vi "HB_ImaqAttributeTree.vi"() -> ()   [LabVIEW 2009, in "HB_IMAQ_Examples.lvlib"]
doc: "The HL Snap VI acquires an image and displays the image in an image control using the high-level acquisition VIs. A snap is appropriate for low-speed or single-capture applications where ease of programming is essential.\n\nIMAQ Init initializes the device. IMAQ Create creates an image buffer. IMAQ Snap acquires an image into the buffer, and an image control displays the image on the front panel. IMAQ Close releases resources associated with the acquisition, and the IMAQ Dispose frees the image buffer. Use this sequence to ensure that the image control displays the image before the memory is disposed."
uses:
  HB_IMAQ_Examples.lvlib
  <vilib>/vision/driver/IMAQdx.llb/IMAQdx Attribute Type.ctl
  lib.lib/HGF_LVC/HGF_IMAQ/HGF_IMAQFactory/HGF_IMAQFactory.lvclass
  lib.lib/HGF_LVC/HGF_IMAQ/HGF_IMAQDevice/HGF_IMAQDevice.lvclass
  lib.lib/HGF_LVC/HGF_BaseClasses/HGF_Factory/HGF_Factory.lvclass
  lib.lib/HGF_LVC/HGF_DeviceBaseClasses/HGF_DeviceBase/HGF_DeviceBase.lvclass
  lib.lib/HGF_LVC/HGF_Auxiliary/HGF_Auxiliary.lvlib
  <vilib>/vision/driver/NI_Vision_Acquisition_Software.lvlib
panel:
  out "Units":string
  out "Tooltip":string
  in  "Attribute Tab Control":T1(tab)
  in  "U32 Value Control":u32(slide) min=1 step=1 scale=1.0..4294967295.0
  in  "DBL Value Control":dbl(slide) min=0.00010395202398217064 max=1000.0 step=1.0 scale=0.00010395202398217064..1000.0
  in  "String Value Control":string
  in  "Enum Value Control":u32(ring) items=["Unicast", "Broadcast", "Multicast"]
  in  "Boolean Value Control":bool=TRUE
  in  "Command Value Control":bool
  in  "Attribute Table":string(tree)
  in  "stop":bool
  out "error out":errorcluster
  out "Attribute Information":T3(array[cluster])
  out "Video Modes":T4(array[cluster])
  in  "cameraName":string="cam0"
  in  "imaqClassName":string="HGF_ImaqDx"
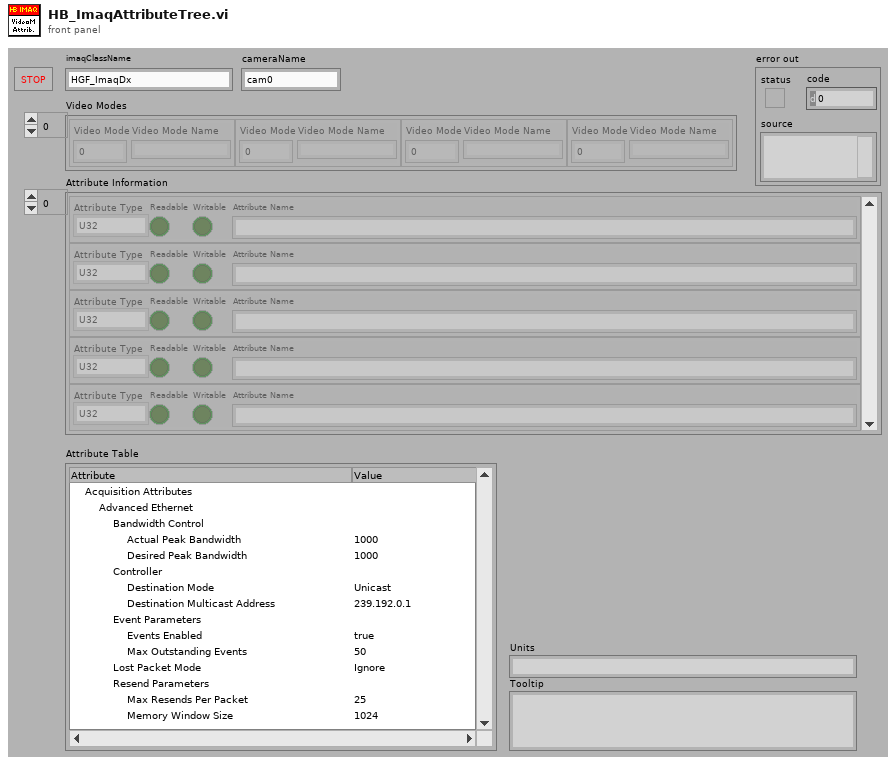
[diagram p1: front panel]
types:
  T1 = enum32{"U32", "DBL", "String", "Enum", "Bool", "Command"}
  T2 = typedef "NI_Vision_Acquisition_Software.lvlib/IMAQdx Attribute Type.ctl" = enum32{"U32", "I64", "DBL", "String", "Enum", "Bool", "Command"}
  T3 = cluster{"Attribute Type":T2, "Readable":bool, "Writable":bool, "Attribute Name":string}[]
  T4 = cluster{"Video Mode":u32, "Video Mode Name":string}[]
  T5 = cluster{"Attribute Tab Control":refnum<vi>, "U32 Value Control":refnum<vi>, "DBL Value Control":refnum<vi>, "String Value Control":refnum<vi>, "Enum Value Control":refnum<vi>, "Boolean Value Control":refnum<vi>, "Command Value Control":refnum<vi>}
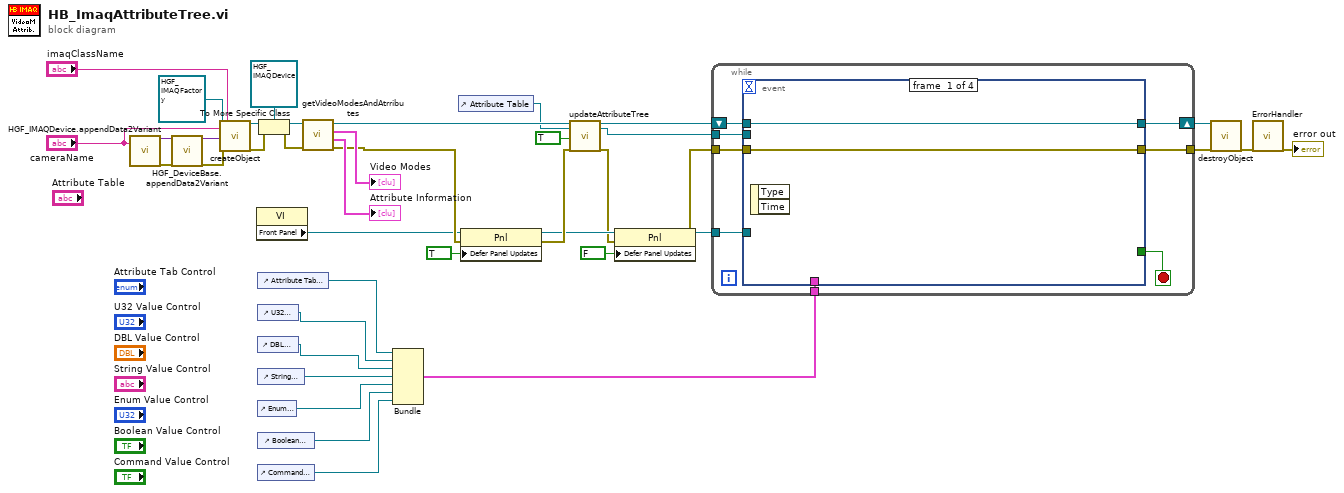
[diagram p0: block diagram]
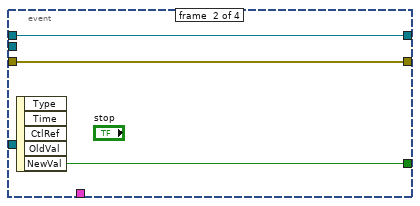
[diagram p2: hidden frame]
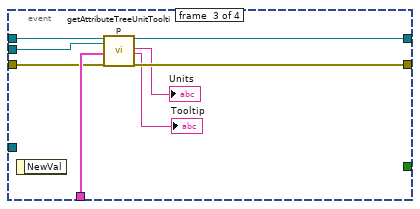
[diagram p3: hidden frame]
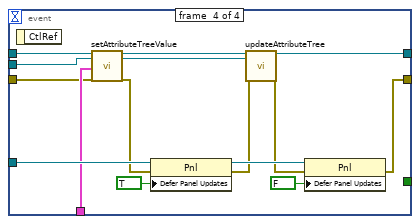
[diagram p4: hidden frame]
diagram:
  n1 = call "HGF_IMAQDevice.appendData2Variant.vi"("cameraName"="cameraName") -> ("dup initData"=w40:variant, "error out"=w39:errorcluster)  [unwired: 5 in, 12 out]
  n2 = call "HGF_DeviceBase.appendData2Variant.vi"("initData"=w40, "error in (no error)"=w39) -> ("dup initData"=w37:variant, "error out"=w38:errorcluster)  [unwired: 16 out]
  n3 = call "createObject.vi"("HGF_Factory"=refnum<class "HGF_IMAQFactory.lvclass"> refnum ("HGF_IMAQ.lvlib:HGF_IMAQFactory.lvclass"), "objectName"="cameraName", "initializationData"=w37, "error in (no error)"=w38, "className"="imaqClassName") -> ("HGF_Object"=w34:refnum<class "HGF_Factory.lvclass">, "error out"=w33:errorcluster)  [unwired: 13 out]
  n4 = property class="VI"() -> ("Front Panel"=w17:refnum<vi>)  [unwired: 2 in, 2 out]
  n5 = control-ref of="Attribute Tab Control"() -> (w4:refnum<vi>)
  n6 = control-ref of="U32 Value Control"() -> (w10:refnum<vi>)
  n7 = control-ref of="DBL Value Control"() -> (w9:refnum<vi>)
  n8 = control-ref of="String Value Control"() -> (w8:refnum<vi>)
  n9 = control-ref of="Enum Value Control"() -> (w7:refnum<vi>)
  n10 = control-ref of="Boolean Value Control"() -> (w6:refnum<vi>)
  n11 = control-ref of="Command Value Control"() -> (w5:refnum<vi>)
  n12 = To More Specific Class(target class=refnum<class "HGF_IMAQDevice.lvclass"> refnum ("HGF_DeviceBaseClasses.lvlib:HGF_IMAQDevice.lvclass"), reference=w34, error in=w33) -> (specific class reference=w29:refnum<class "HGF_IMAQDevice.lvclass">, error out=w28:errorcluster)
  n13 = call "getVideoModesAndAtrributes.vi"("error in (no error)"=w28, "HGF_IMAQDevice in"=w29) -> ("error out"=w21:errorcluster, "Attribute Information"=→"Attribute Information":T3, "Video Modes"=→"Video Modes":T4, "HGF_IMAQDevice out"=w25:refnum<class "HGF_IMAQDevice.lvclass">)  [unwired: 5 in, 1 out]
  n14 = Bundle("Attribute Tab Control"=w4, "U32 Value Control"=w10, "DBL Value Control"=w9, "String Value Control"=w8, "Enum Value Control"=w7, "Boolean Value Control"=w6, "Command Value Control"=w5) -> (w3:T5)  [unwired: 1 out]
  n15 = control-ref of="Attribute Table"() -> (w24:refnum<vi>)
  n16 = property class="Pnl"(reference=w17, error in=w21, "Defer Panel Updates"=TRUE) -> (reference out=w19:refnum<vi>, error out=w20:errorcluster)
  n17 = call "updateAttributeTree.vi"("HGF_IMAQDevice"=w25, "Tree Control In"=w24, "Flush Tree?"=TRUE, "error in (no error)"=w20) -> ("dup HGF_IMAQDevice"=w14:refnum<class "HGF_IMAQDevice.lvclass">, "Tree Control Out"=w2:refnum<vi>, "error out"=w18:errorcluster)  [unwired: 13 in]
  n18 = property class="Pnl"(reference=w19, error in=w18, "Defer Panel Updates"=FALSE) -> (reference out=w1:refnum<vi>, error out=w13:errorcluster)
  n19 = while {
    tunnel: w13 -> [w46]
    tunnel: [w45] -> w12
    shift-right: [w48] -> w11
    shift-left: w14 -> [w47]
    tunnel: w3 -> [w43]
    tunnel: w2 -> [w42]
    tunnel: w1 -> [w41]
    stop <- w44 stop-if-true
    n20 = event shown="[3] \"Command Value Control\", \"Boolean Value Control\", \"Enum Value Control\", \"String Value Control\", \"DBL Value Control\", \"U32 Value Control\": Value Change;  \"DBL Value Control\", \"U32 Value Control\": Mouse Up" {
      selector: _ -> [_ _ _ _]
      dyn-events: _ -> [_ _ _ _]
      timeout: _ -> [_ _ _ _]
      tunnel: [w50 w52 w60 w66] -> w48
      tunnel: w47 -> [w50 w52 w61 w73]
      tunnel: w46 -> [w49 w51 w57 w69]
      tunnel: [w49 w51 w56 w62] -> w45
      tunnel: [_ w53 _ _] -> w44
      tunnel: w43 -> [_ _ w58 w71]
      tunnel: w42 -> [_ _ w59 w70]
      tunnel: w41 -> [_ _ _ w74]
      event #0 {
        n21 = event-data() -> ()  [unwired: 1 in, 2 out]
      }
      event #1 {
        n22 = event-data() -> ("NewVal"=w53:bool)  [unwired: 1 in, 4 out]
      }
      event #2 {
        n23 = event-data() -> ()  [unwired: 1 in, 1 out]
        n24 = call "getAttributeTreeUnitTooltip.vi"("HGF_IMAQDevice"=w61, "Tree Control In"=w59, "Tab Control Ref In"=w58, "error in (no error)"=w57) -> ("dup HGF_IMAQDevice"=w60:refnum<class "HGF_IMAQDevice.lvclass">, "Units"=→"Units":string, "Tooltip"=→"Tooltip":string, "error out"=w56:errorcluster)  [unwired: 11 in, 1 out]
      }
      event #3 {
        n25 = event-data() -> ()  [unwired: 1 in, 1 out]
        n26 = call "setAttributeTreeValue.vi"("HGF_IMAQDevice"=w73, "Tree Control In"=w70, "Tab Control Ref In"=w71, "error in (no error)"=w69) -> ("dup HGF_IMAQDevice"=w67:refnum<class "HGF_IMAQDevice.lvclass">, "Tree Control Out"=w63:refnum<vi>, "error out"=w68:errorcluster)  [unwired: 13 in]
        n27 = property class="Pnl"(reference=w74, error in=w68, "Defer Panel Updates"=TRUE) -> (reference out=w72:refnum<vi>, error out=w65:errorcluster)
        n28 = call "updateAttributeTree.vi"("HGF_IMAQDevice"=w67, "Tree Control In"=w63, "error in (no error)"=w65) -> ("dup HGF_IMAQDevice"=w66:refnum<class "HGF_IMAQDevice.lvclass">, "error out"=w64:errorcluster)  [unwired: 14 in, 1 out]
        n29 = property class="Pnl"(reference=w72, error in=w64, "Defer Panel Updates"=FALSE) -> (error out=w62:errorcluster)  [unwired: 1 out]
      }
    }
  }
  n30 = call "destroyObject.vi"("HGF_Factory"=w11, "error in (no error)"=w12) -> ("error out"=w30:errorcluster)  [unwired: 17 out]
  n31 = call "ErrorHandler.vi"("error in (no error)"=w30) -> ("error out"=→"error out":errorcluster)  [unwired: 6 in, 12 out]
